vi "Orb_Shutdown.vi"(9 "error in (no error)":errorcluster) -> (6 "error out":errorcluster)   [LabVIEW 2009]
uses:
  Orb_Global.vi
  lib/lvrtc.dll
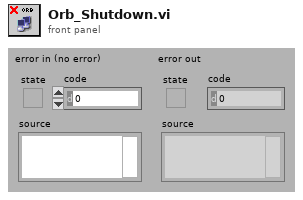
[diagram p1: front panel]
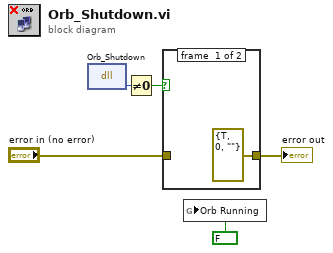
[diagram p0: block diagram]
diagram:
  n1 = dll-call lib="C:/Ohana/LV2009/OhanaOS-LV81/Instruments/RTC/Api/lib/lvrtc.dll" fn="Orb_Shutdown"() -> ("return type"=w4:i32)  [unwired: 3 in, 2 out]
  n2 = Not Equal To 0?(x=w4) -> (x != 0?=w1:bool)
  n3 = case shown="True" w1 {
    tunnel: [errorcluster {"status"=TRUE, "code"=0, "source"=""} ("error in (no error)") w7] -> w3
    tunnel: "error in (no error)" -> [_ w7]
    frame #0 {
    }
    frame #1 {
    }
  }
  "error out" <- w3
  n4 = global write "Orb_Global.vi" "Orb Running"(FALSE ("Orb Running")) -> ()
